vi "poly_error_bypass_out.vi"(9 "Error in":errorcluster) -> (1 "No error":errorcluster, 2 "Error out":errorcluster)   [LabVIEW 2015]
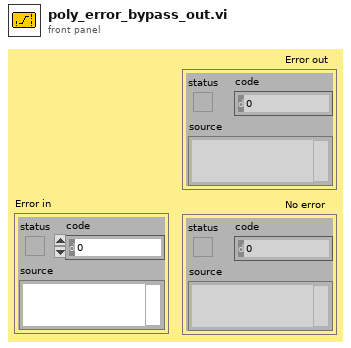
[diagram p1: front panel]
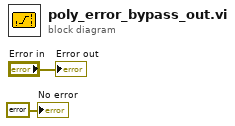
[diagram p0: block diagram]
diagram:
  "Error out" <- "Error in"
  "No error" <- errorcluster {"status"=FALSE, "code"=0, "source"=""} ("error constant")
